vi "lasttime_wr.vi"(4 "error in":errorcluster, 5 "name":string="lasttime.txt", 6 "time stamp":timestamp, 7 "start Path":path=path "C:/skill/My Application/vi.lib") -> (0 "error out":errorcluster, 3 "file path":path)   [LabVIEW 2010]
uses:
  user32.dll
panel:
  in  "stop_qw":bool caption="Остановить"
  in  "OK Button":bool caption="Проверить"
  out "standard output":string
  in  "Tab Control":enum32{"Error In", "Error Out"}(tab)
  out "date/time string":string
  # "Время и дата для\nскриптового watchdog-а."
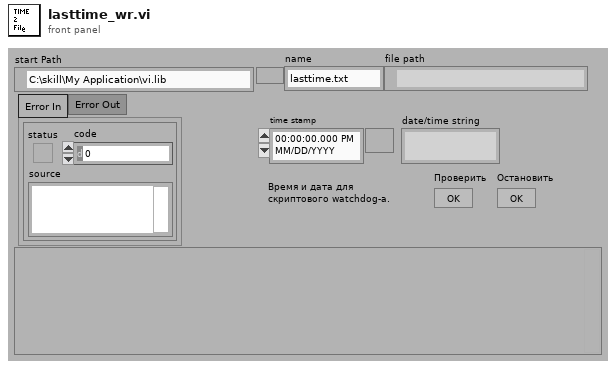
[diagram p1: front panel]
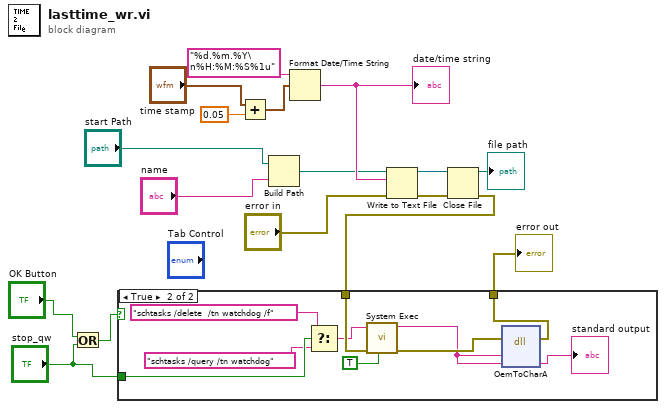
[diagram p0: block diagram]
diagram:
  n1 = Or(x="OK Button", y="stop_qw") -> (x .or. y?=w1:bool)
  n2 = Add(x="time stamp", y=0.05) -> (x+y=w6:timestamp)
  n3 = Build Path(base path="start Path", name or relative path="name") -> (appended path=w11:path)
  n4 = Format Date/Time String(time format string (%c)="%d.%m.%Y\n%H:%M:%S%1u", seconds (now)=w6) -> (date/time string=w14:string)  [unwired: 1 in]
  "date/time string" <- w14
  n5 = Write to Text File(file (use dialog)=w11, text=w14, error in="error in") -> (refnum out=w12:refnum<file>, error out=w13:errorcluster)  [unwired: 1 in, 1 out]
  n6 = Close File(refnum=w12, error in=w13) -> (path=→"file path":path, error out=w5:errorcluster)
  n7 = case shown="True" w1 {
    tunnel: w5 -> [w18 w24]
    tunnel: [w18 w23] -> w4
    tunnel: "stop_qw" -> [_ w22]
    frame False {
    }
    frame True {
      n8 = Select(t="schtasks /delete  /tn watchdog /f", s=w22, f="schtasks /query /tn watchdog") -> (s? t:f=w19:string)
      n9 = call <vilib>:"System Exec.vi"("run minimized? (F)"=TRUE, "error in (no error)"=w24, "command line"=w19) -> ("error out"=w27:errorcluster, "standard output"=w26:string)  [unwired: 5 in, 2 out]
      n10 = dll-call lib="user32.dll" fn="OemToCharA"(error in=w27, "src"=w26, "dst"=w26) -> (error out=w23:errorcluster, "dst"=→"standard output":string)  [unwired: 4 in, 1 out]
    }
  }
  "error out" <- w4
